vi "Get Property.vi"(10 "Ctl Ref":refnum<vi>, 11 "CaptionUIP In":refnum<class "CaptionUIP.lvclass">) -> (0 "Error Out":errorcluster, 3 "CaptionUIP Out":refnum<class "CaptionUIP.lvclass">)   [LabVIEW 2015, in "CaptionUIP.lvclass"]
doc: "Modify this method to implement functionality for extracting the property from VI Server Control to be stored inside UIP."
uses:
  CaptionUIP.lvclass
  CaptionUIP.lvclass/CaptionUIP.ctl
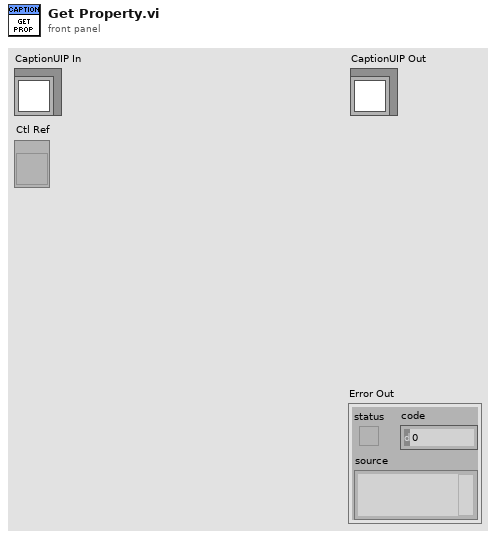
[diagram p1: front panel]
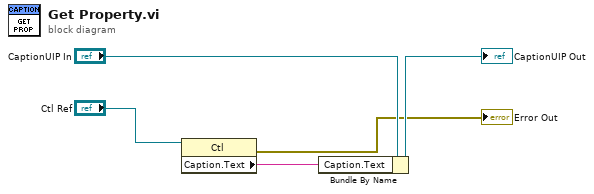
[diagram p0: block diagram]
diagram:
  n1 = property class="Ctl"(reference="Ctl Ref") -> (error out=→"Error Out":errorcluster, "Caption.Text"=w2:string)  [unwired: 1 in, 1 out]
  n2 = Bundle By Name(cluster="CaptionUIP In", "Caption.Text"=w2) -> (→"CaptionUIP Out":refnum<class "CaptionUIP.lvclass">)
